vi "List API.vi"(8 "error in (no error)":errorcluster, 11 "SMOFacade in":refnum<class "SMOFacade.lvclass">) -> (0 "error out":errorcluster, 2 "Public API":string[](array[string]), 3 "SMOFacade out":refnum<class "SMOFacade.lvclass">)   [LabVIEW 2013, in "SMOFacade.lvclass"]
uses:
  SMOFacade.lvclass
  SMOFacade.lvclass/SMOFacade.ctl
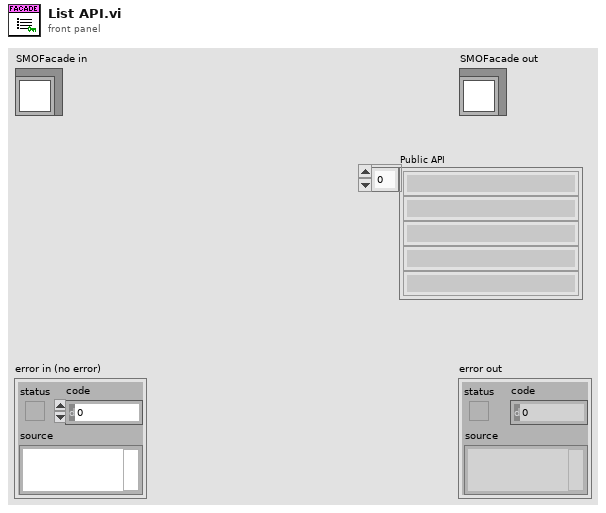
[diagram p1: front panel]
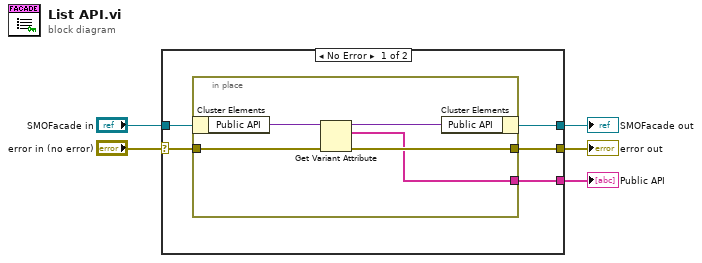
[diagram p0: block diagram]
diagram:
  n1 = case shown="No Error" "error in (no error)" {
    selector: "error in (no error)" -> [w8 w17]
    tunnel: [w7 w17] -> w4
    tunnel: [w9 w16] -> w2
    tunnel: "SMOFacade in" -> [w10 w16]
    tunnel: [w6 _] -> w1
    frame No Error {
      n2 = in-place {
        in-place-border: w8 -> [w13]
        in-place-border: [w12] -> w7
        in-place-border: [w11] -> w6
        n3 = in-place-cluster #1(w10) -> ("Public API"=w15:variant)
        n4 = Get Variant Attribute(Variant=w15, error in=w13) -> (duplicate Variant=w14:variant, names=w11:string[], error out=w12:errorcluster)  [unwired: 2 in, 1 out]
        n5 = in-place-cluster #1("Public API"=w14) -> (w9:refnum<class "SMOFacade.lvclass">)
      }
    }
    frame Error {
    }
  }
  "error out" <- w4
  "SMOFacade out" <- w2
  "Public API" <- w1
